vi "Request Identities.vi"(5 "Username":string, 6 "Password":string, 7 "Address":string, 8 "Error In":errorcluster) -> (0 "Error Out":errorcluster)   [LabVIEW 2018, in "Tests.lvlib" / "Agent.lvlib"]
uses:
  Agent.lvlib
  <vilib>/addons/_JKI Toolkits/Caraya/classes/Test/Test.lvclass
  <vilib>/addons/_JKI Toolkits/Caraya/classes/Assert/Assert.lvclass
  src/Toolkit/Agent/Agent.lvclass
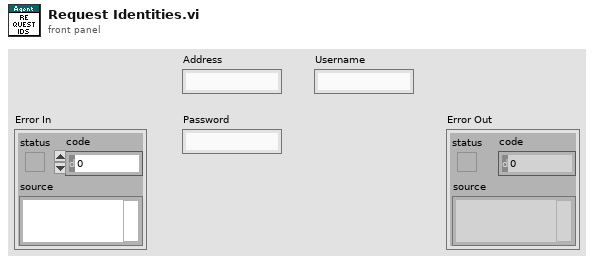
[diagram p1: front panel]
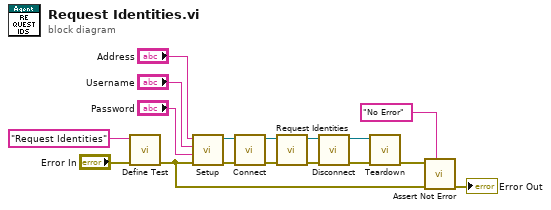
[diagram p0: block diagram]
diagram:
  n1 = call <vilib>:"Define Test.vi"("error in (no error)"="Error In", "Label (VI Title)"="Request Identities") -> ("error out"=w14:errorcluster)  [unwired: 9 in]
  n2 = call "Setup.vi"("Error In"=w14, "Password"="Password", "Username"="Username", "Address"="Address") -> ("Error Out"=w12:errorcluster, "Agent"=w13:refnum<class "Agent.lvclass">)  [unwired: 6 in]
  n3 = call "Connect.vi"("Error In"=w12, "Agent In"=w13) -> ("Error Out"=w10:errorcluster, "Agent Out"=w11:refnum<class "Agent.lvclass">)  [unwired: 8 in]
  n4 = call "Request Identities.vi"("Error In"=w10, "Agent In"=w11) -> ("Error Out"=w2:errorcluster, "Agent Out"=w3:refnum<class "Agent.lvclass">)  [unwired: 8 in]
  n5 = call "Disconnect.vi"("Error In"=w2, "Agent In"=w3) -> ("Error Out"=w8:errorcluster, "Agent Out"=w7:refnum<class "Agent.lvclass">)  [unwired: 8 in]
  n6 = call "Teardown.vi"("Error In"=w8, "Agent"=w7) -> ("Error Out"=w9:errorcluster)  [unwired: 9 in]
  n7 = call <vilib>:"Assert Not Error.vi"("Label"="No Error", "error in (no error)"=w14, "Not Error?"=w9) -> ("error out"=→"Error Out":errorcluster)  [unwired: 8 in]
